vi "cluster_v41.vi"() -> ()   [LabVIEW 2010]
panel:
  in  "Reset Signal 2":bool=TRUE
  in  "Faza 2":dbl(slide)=145.41176470588238 scale=0.0..360.0
  in  "Frecventa 2":dbl(knob)=71.59018489970538 min=0.0 max=10.0 step=1.0 scale=0.0..100.0
  in  "Amplitudine 2":dbl(slide)=7.737226277372262 scale=0.0..10.0 scale format="%#1_6g"
  in  "Reset Signal":bool=TRUE
  in  "stop":bool
  in  "Faza":dbl(slide)=46.58823529411765 scale=0.0..360.0
  in  "Frecventa":dbl(knob)=28.751924365486083 min=0.0 max=10.0 step=1.0 scale=0.0..100.0
  out "Waveform Graph":dynamicdata(graph)=[{"t0"=timestamp(63.64804172515869 s since 1904-01-01), "dt"=0.001, "Y"=[4.128190795070173, 4.762711581857739, 5.242219981134554, 5.5511093913825835, 5.679326362138502, 5.6226978045190785, 5.383066813107518, 4.968232678593972, 4.391697043584066, 3.6722244634643433, 2.833231674788351, 1.9020254487182084, 0.9089138351719219, -0.11378027590964374, -1.132771170469015, -2.1148936633584987, -3.0281825285016883, -3.8429128738828426, -4.532567600189028, -5.074700455144536, -5.451666593633243, -5.651196866005093, -5.666797143155391, -5.4979596815087906, -5.150179648593555, -4.634776271346731, -3.9685244282519294, -3.1731086759123586, -2.274417479903701, -1.3017006206365214, -0.286617198212815, 0.7377947790547011, 1.7381936855685978, 2.682019451230868, 3.5385532968723585, 4.279917541026394, 4.881982937248752, 5.325154010797362, 5.595006834250683, 5.682758484326233, 5.585552900447512, 5.306553841195614, 4.854841913183937, 4.24511902376603, 3.497229876780076, 2.6355160852494763, 1.6880239227896512, 0.6855914991047646, -0.3391549306471991, -1.352862855414746, -2.3225390353268462, -3.21662333553656, -4.0060159166710205, -4.665024349830882, -5.172199830305209, -5.5110352736812525, -5.670502573354574, -5.645411533272473, -5.4365787936957455, -5.050801251937145, -4.500634843154255, -3.8039858812373546, -2.983528260456047, -2.065965486253145, -1.0811615539337571, -0.061168962616309726, 0.9608145002401244, 1.9515262501075692, 2.8787215056167597, 3.712222762256892, 4.424901982235984, 4.993563533083001, 5.399699137912546, 5.630090265920104, 5.677238357052252, 5.539608878291945, 5.221681268237947, 4.7338031444276565, 4.09185351853044, 3.3167259807756504, 2.433648674456789, 1.47136319336057, 0.461189126617663, -0.5639953026849504, -1.5708233278863666, -2.5265256298042638, -3.3999968826124687, -4.162808141582179, -4.790132122415235, -5.2615512570224485, -5.561722225885584, -5.680875338410271, -5.6151325078943755, -5.366633471952647, -4.943466150290795, -4.3594034064803076, -3.6334547813716265, -2.7892477879170086, -1.8542589044543785, -0.8589192953804297], "attributes"=variant("NI_ChannelName"=variant(string "Sine"), "NI_ExpIsRelativeTime"=variant(bool TRUE), "NI_ExpStartTimeStamp"=variant(timestamp timestamp(3685618368.2497225 s since 1904-01-01)), "NI_ExpTimeStamp"=variant(timestamp timestamp(3685618431.897764 s since 1904-01-01)), "NI_ExpXDimension"=variant(string "t"))}, {"t0"=timestamp(63.64804172515869 s since 1904-01-01), "dt"=0.001, "Y"=[4.392227730753761, 1.1857903315880973, -2.2565533724520277, -5.249968498086377, -7.1989319731222725, -7.7157084960623274, -6.697488289557963, -4.346840526308762, -1.131413333574164, 2.30910216667911, 5.2902348020128045, 7.218905032471184, 7.711414783218821, 6.6697820144983995, 4.301233696339166, 1.0769791705353327, -2.3615342927718004, -5.330233815113498, -7.238513354306681, -7.706731448647336, -6.641738746543647, -4.255409545144825, -1.0224905927753087, 2.4138471015799583, 5.3699635164253685, 7.257755947911965, 7.701658728974857, 6.613359902588905, 4.209370388005803, 0.9679503533471219, -2.4660379499819842, -5.409421898592404, -7.276631841048757, -7.696196880502198, -6.584646916484441, -4.163118551065426, -0.9133612079140204, 2.518104201018372, 5.448606967967066, 7.295140080006456, 7.69034617919101, 6.555601238963182, 4.116656371212717, 0.8587259146102505, -2.5700432240249325, -5.487516744711049, -7.313279729650287, -7.684106920649882, -6.526224337567376, -4.069986195964361, -0.8040472339016865, 2.621852394765717, 5.52614926289528, 7.331049873468591, 7.6774794201193615, 6.496517696574484, 4.023110383346061, 0.7493279284463747, -2.6735290955656046, -5.56450257059928, -7.348449613619089, -7.6704640124560655, -6.46648281692215, -3.9760313017734283, -0.6945707629549314, 2.72507071544256, 5.602574730009757, 7.365478070974288, 7.66306105211573, 6.436121216132398, 3.9287513299322936, 0.6397785040508692, -2.7764746502395554, -5.64036381751854, -7.38213438516586, -7.65527091313533, -6.405434428234928, -3.881272856658542, -0.5849539201308034, 2.8277383027561482, 5.677867923819743, 7.398417714628145, 7.647093989114151, 6.3744240036896365, 3.8335982808174007, 0.5300997812245825, -2.878859082879699, -5.715085154006264, -7.414327236640647, -7.638530693193933, -6.343091509308259, -3.7857300111822463, -0.4752188588553314, 2.9298344077162484, 5.752013627665494, 7.4298621473696205, 7.629581458037969, 6.311438528175216, 3.737670466312898, 0.4203139258994139], "attributes"=variant("NI_ChannelName"=variant(string "Sine"), "NI_ExpIsRelativeTime"=variant(bool TRUE), "NI_ExpStartTimeStamp"=variant(timestamp timestamp(3685618368.2497225 s since 1904-01-01)), "NI_ExpTimeStamp"=variant(timestamp timestamp(3685618431.897764 s since 1904-01-01)), "NI_ExpXDimension"=variant(string "t"))}]
  in  "Amplitudine":dbl(slide)=5.682819383259912 scale=0.0..10.0 scale format="%#1_6g"
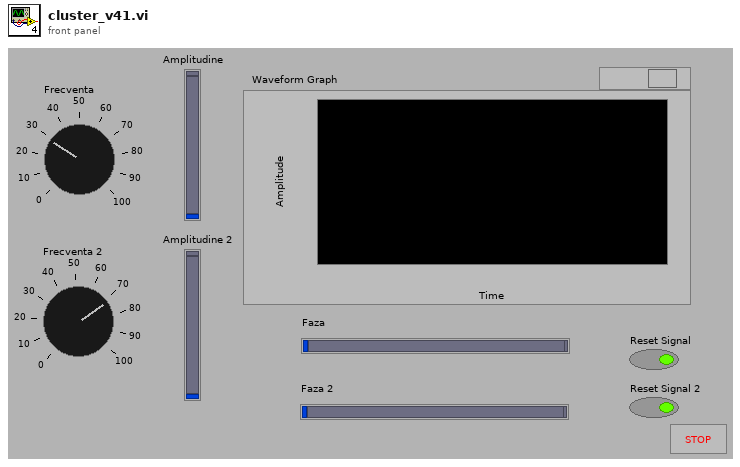
[diagram p1: front panel]
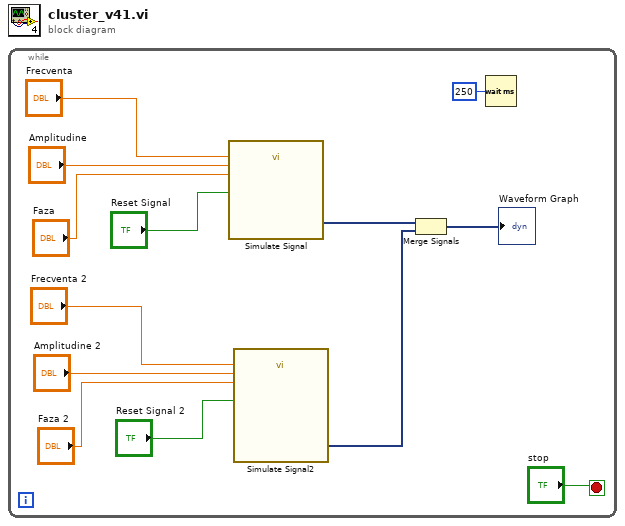
[diagram p0: block diagram]
diagram:
  n1 = while {
    stop <- "stop" stop-if-true
    n2 = call "Simulate Signal"("Reset Signal"="Reset Signal", "Frequency"="Frecventa", "Amplitude"="Amplitudine", "Phase"="Faza") -> ("Sine"=w2:dynamicdata)  [unwired: 10 in, 1 out]
    n3 = call "Simulate Signal2"("Reset Signal"="Reset Signal 2", "Frequency"="Frecventa 2", "Amplitude"="Amplitudine 2", "Phase"="Faza 2") -> ("Sine"=w1:dynamicdata)  [unwired: 10 in, 1 out]
    n4 = Merge Signals(w2, w1) -> (→"Waveform Graph":dynamicdata)
    n5 = Wait (ms)(milliseconds to wait=u32 250) -> ()  [unwired: 1 out]
  }
